vi "getLifetime.vi"(8 "error in (no error)":errorcluster, 10 "dt (ns)":dbl=0.4, 11 "LaguerreDeconEngineClass in":refnum<class "LaguerreDeconEngineClass.lvclass">) -> (0 "error out":errorcluster, 2 "lifetime (ns)":dbl, 3 "LaguerreDeconEngineClass out":refnum<class "LaguerreDeconEngineClass.lvclass">)   [LabVIEW 2020, in "LaguerreDeconEngineClass.lvclass"]
uses:
  LaguerreDeconEngineClass.lvclass
panel:
  out "Waveform Graph":dbl[](graph)
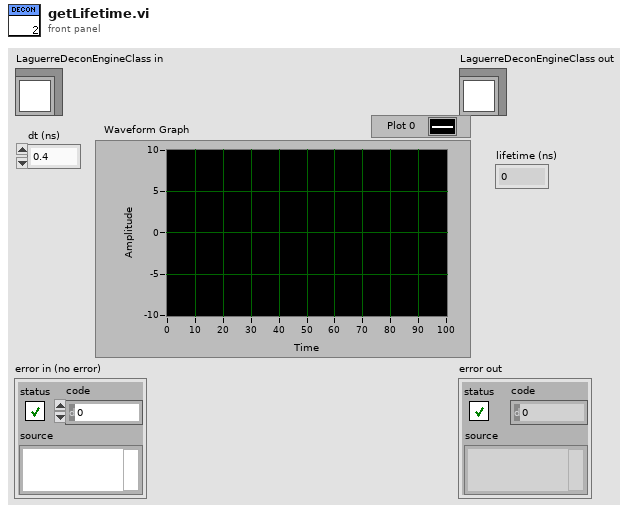
[diagram p1: front panel]
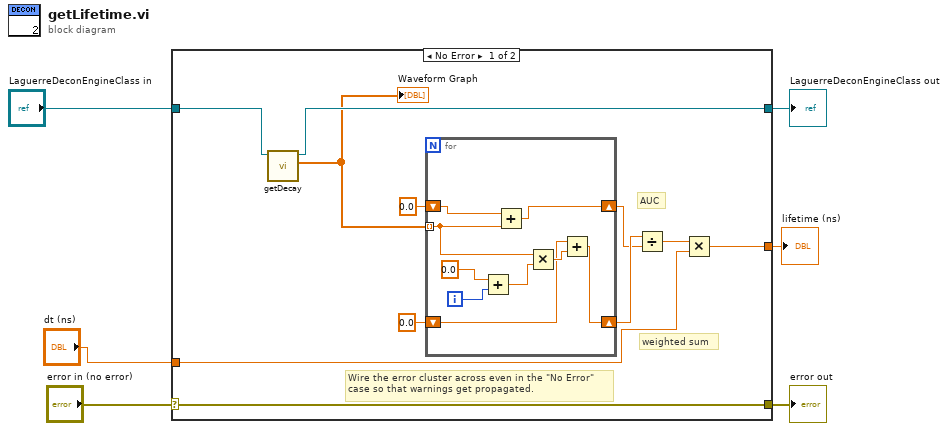
[diagram p0: block diagram]
diagram:
  n1 = case shown="No Error" "error in (no error)" {
    selector: "error in (no error)" -> [w17 w28]
    tunnel: [w17 w28] -> w5
    tunnel: [w15 w27] -> w3
    tunnel: "LaguerreDeconEngineClass in" -> [w16 w27]
    tunnel: "dt (ns)" -> [w9 _]
    tunnel: [w8 _] -> w1
    frame No Error {
      # "weighted sum"
      # "AUC"
      # "Wire the error cluster across even in the \"No Error\"\ncase so that warnings get propagated."
      n2 = call "getDecay.vi"("LaguerreDeconClass in"=w16) -> ("Decay"=w7:dbl[], "LaguerreDeconClass out"=w15:refnum<class "LaguerreDeconEngineClass.lvclass">)  [unwired: 8 in, 1 out]
      "Waveform Graph" <- w7
      n3 = for {
        tunnel: w7 -> [w20] mode=indexing
        shift-right: [w22] -> w12
        shift-left: 0.0 -> [w23]
        shift-right: [w18] -> w11
        shift-left: 0.0 -> [w21]
        i -> [w19]
        n4 = Add(x=0.0, y=w19) -> (x+y=w25:dbl)
        n5 = Add(x=w21, y=w20) -> (x+y=w18:dbl)
        n6 = Multiply(x=w20, y=w25) -> (x*y=w24:dbl)
        n7 = Add(x=w23, y=w24) -> (x+y=w22:dbl)
      }
      n8 = Divide(x=w12, y=w11) -> (x/y=w10:dbl)
      n9 = Multiply(x=w10, y=w9) -> (x*y=w8:dbl)
    }
    frame Error {
    }
  }
  "error out" <- w5
  "LaguerreDeconEngineClass out" <- w3
  "lifetime (ns)" <- w1
